vi "UTEXKeyboardControl.vi"(8 "PlatMods":T1, 10 "Char":i16, 11 "UT340 Controls":refnum<vi>) -> ()   [LabVIEW 2022 SP3]
uses:
  Controls/UTEX Controls Simple.ctl
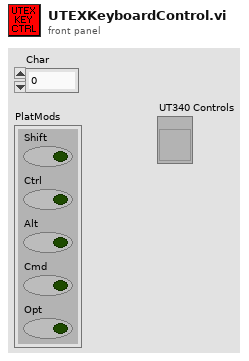
[diagram p1: front panel]
types:
  T1 = cluster{"Shift":bool, "Ctrl":bool, "Alt":bool, "Cmd":bool, "Opt":bool}
  T2 = typedef "UTEX Controls Simple.ctl" = cluster{"PE Gain (dB)":i16, "Voltage":i16}
  T3 = typedef "LVStringsAndValuesArrayTypeDef_U16.ctl" = cluster{"String":string, "Value":u16}[]
  T4 = typedef "LVStringsAndValuesArrayTypeDef_I32.ctl" = cluster{"String":string, "Value":i32}[]
  T5 = typedef "LVStringsAndValuesArrayTypeDef_DBL.ctl" = cluster{"String":string, "Value":dbl}[]
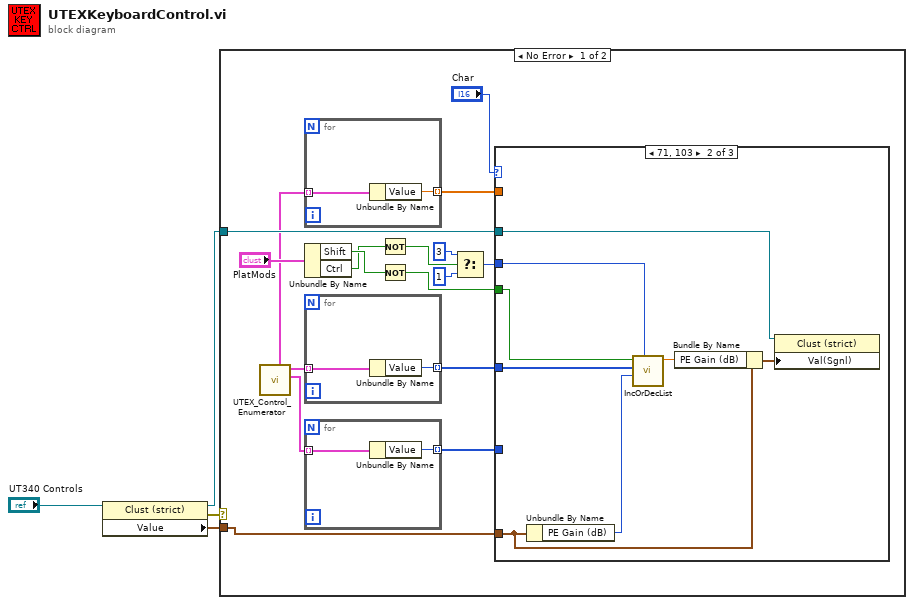
[diagram p0: block diagram]
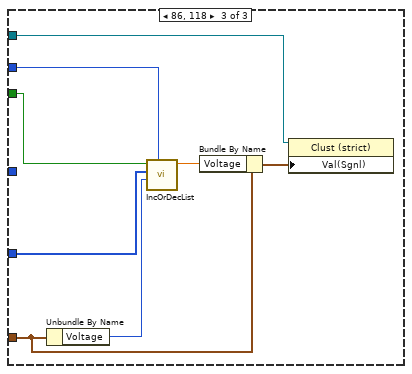
[diagram p3: hidden frame]
diagram:
  n1 = property on="Property Node" class="Clust (strict)"(reference="UT340 Controls") -> (reference out=w3:refnum<vi>, error out=w2:errorcluster, "Value"=w4:T2)  [unwired: 1 in]
  n2 = case shown="No Error" w2 {
    tunnel: w4 -> [w19 _]
    tunnel: w3 -> [w18 _]
    frame No Error {
      n3 = call "UTEX_Control_Enumerator.vi"() -> ("Voltage (V)"=w12:T3, "Gain (dB)"=w11:T4, "Pulse Width (ns)"=w10:T5)  [unwired: 7 in, 2 out]
      n4 = for {
        tunnel: w10 -> [w23] mode=indexing
        tunnel: [w22] -> w14 mode=indexing
        n5 = Unbundle By Name(w23) -> ("Value"=w22:dbl)
      }
      n6 = Unbundle By Name("PlatMods") -> ("Shift"=w17:bool, "Ctrl"=w9:bool)
      n7 = for {
        tunnel: w11 -> [w25] mode=indexing
        tunnel: [w24] -> w15 mode=indexing
        n8 = Unbundle By Name(w25) -> ("Value"=w24:i32)
      }
      n9 = for {
        tunnel: w12 -> [w43] mode=indexing
        tunnel: [w42] -> w16 mode=indexing
        n10 = Unbundle By Name(w43) -> ("Value"=w42:u16)
      }
      n11 = Not(x=w9) -> (.not. x?=w8:bool)
      n12 = Not(x=w17) -> (.not. x?=w13:bool)
      n13 = Select(t=3, s=w8, f=1) -> (s? t:f=w6:i32)
      n14 = case shown="71, 103" "Char" {
        tunnel: w19 -> [_ w33 w41]
        tunnel: w18 -> [_ w31 w39]
        tunnel: w13 -> [_ w29 w37]
        tunnel: w16 -> [_ _ w36]
        tunnel: w15 -> [_ w28 _]
        tunnel: w14 -> [_ _ _]
        tunnel: w6 -> [_ w26 w34]
        frame Default {
        }
        frame 71, 103 {
          n15 = Unbundle By Name(w33) -> ("PE Gain (dB)"=w27:i16)
          n16 = call "IncOrDecList.vi"("Step Size?"=w26, "Input"=w27, "Vals"=w28, "Shift"=w29) -> ("Output"=w30:dbl)  [unwired: 7 in]
          n17 = Bundle By Name(cluster=w33, "PE Gain (dB)"=w30) -> (w32:T2)
          n18 = property class="Clust (strict)"(reference=w31, "Val(Sgnl)"=w32) -> ()  [unwired: 1 in, 2 out]
        }
        frame 86, 118 {
          n19 = Unbundle By Name(w41) -> ("Voltage"=w35:i16)
          n20 = call "IncOrDecList.vi"("Step Size?"=w34, "Input"=w35, "Vals"=w36, "Shift"=w37) -> ("Output"=w38:dbl)  [unwired: 7 in]
          n21 = Bundle By Name(cluster=w41, "Voltage"=w38) -> (w40:T2)
          n22 = property class="Clust (strict)"(reference=w39, "Val(Sgnl)"=w40) -> ()  [unwired: 1 in, 2 out]
        }
      }
    }
    frame Error {
    }
  }
